vi "AUTOFLIM_move_to_emitter.vi"(0 "Mesh":dbl, 1 "YScale.Offset":dbl, 3 "XScale.Offset":dbl, 5 "cent":i32[][](array[numeric]), 7 "Drift":dbl[](array[numeric]), 9 "System no.":i32, 11 "error in (no error)":errorcluster, 12 "Z":dbl, 14 "Emitter # in":i32) -> (4 "Numeric 2":dbl, 6 "Numeric":dbl, 10 "Emitter # out":i32, 15 "error out":errorcluster)   [LabVIEW 2023]
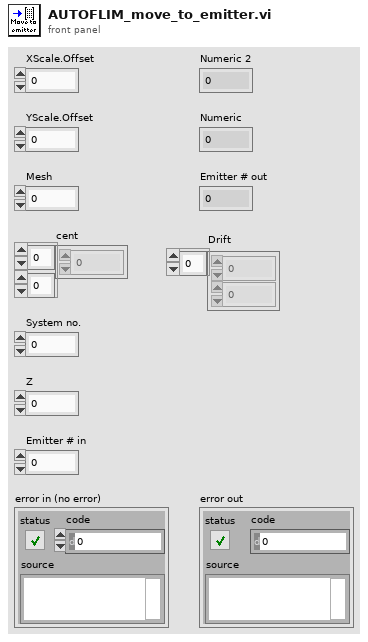
[diagram p1: front panel]
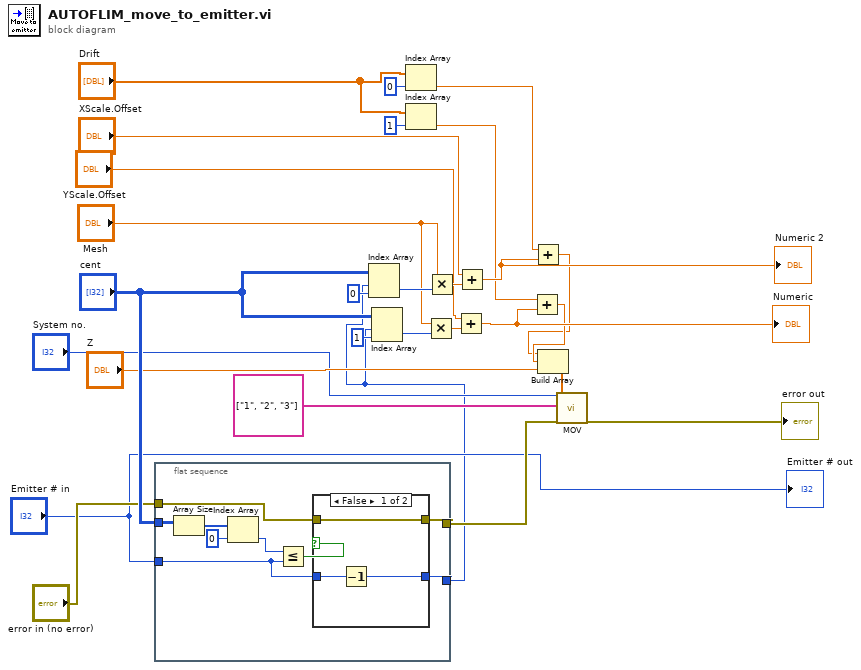
[diagram p0: block diagram]
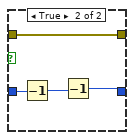
[diagram p2: hidden frame]
diagram:
  n1 = flat-sequence {
    tunnel: "error in (no error)" -> [w37]
    tunnel: [w36] -> w13
    tunnel: "cent" -> [w35]
    tunnel: "Emitter # in" -> [w30]
    tunnel: [w29] -> w10
    frame #0 {
      n2 = Array Size(array=w35) -> (size(s)=w34:i32[])
      n3 = Index Array(array=w34, index=0) -> (element=w32:i32)
      n4 = Less Or Equal?(x=w32, y=w30) -> (x <= y?=w31:bool)
      n5 = case shown="False" w31 {
        tunnel: w37 -> [w40 w44]
        tunnel: [w40 w44] -> w36
        tunnel: w30 -> [w39 w43]
        tunnel: [w38 w41] -> w29
        frame False {
          n6 = Decrement(x=w39) -> (x-1=w38:i32)
        }
        frame True {
          n7 = Decrement(x=w43) -> (x-1=w42:i32)
          n8 = Decrement(x=w42) -> (x-1=w41:i32)
        }
      }
    }
  }
  n9 = Index Array(array="cent", index (row)=w10, index (col)=0 ("disabled index (col)")) -> (element=w26:i32)
  n10 = Index Array(array="cent", index (row)=w10, index (col)=1 ("disabled index (col)")) -> (element=w27:i32)
  n11 = Index Array(array="Drift", index=0) -> (element=w5:dbl)
  n12 = Index Array(array="Drift", index=1) -> (element=w3:dbl)
  n13 = Multiply(x="Mesh", y=w27) -> (x*y=w24:dbl)
  n14 = Multiply(x="Mesh", y=w26) -> (x*y=w23:dbl)
  n15 = Add(x="YScale.Offset", y=w24) -> (x+y=w4:dbl)
  "Numeric" <- w4
  n16 = Add(x="XScale.Offset", y=w23) -> (x+y=w6:dbl)
  "Numeric 2" <- w6
  n17 = Add(x=w3, y=w4) -> (x+y=w2:dbl)
  n18 = Add(x=w5, y=w6) -> (x+y=w1:dbl)
  n19 = Build Array(w1, w2, "Z") -> (w17:dbl[])
  n20 = call "MOV.vi"("System no."="System no.", "Axes to move"=string[] ["1", "2", "3"], "Position values"=w17, "error in"=w13) -> ("error out"=→"error out":errorcluster)  [unwired: 1 in, 14 out]
  "Emitter # out" <- "Emitter # in"
